vi "Unformat Mapping.vi"(3 "Formatted Mapping":string) -> (1 "Mapping Path":string)   [LabVIEW 2016, in "System Mapping Tool.lvlib"]
uses:
  System Mapping Tool.lvlib
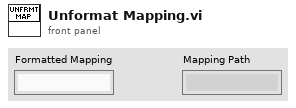
[diagram p1: front panel]
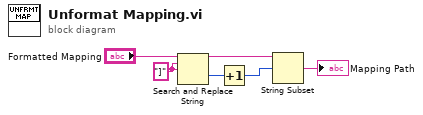
[diagram p0: block diagram]
diagram:
  w3 = "]" ("search string")
  n1 = Search and Replace String(input string="Formatted Mapping", search string=w3, replace string=w3) -> (result string=w4:string, offset past replacement=w6:i32)  [unwired: 5 in, 2 out]
  n2 = Increment(x=w6) -> (x+1=w5:i32)
  n3 = String Subset(string=w4, offset (0)=w5) -> (substring=→"Mapping Path":string)  [unwired: 1 in]
